vi "Handle Scroll.vi"(8 "error in (no error)":errorcluster, 9 "OldVal":i32, 10 "NewVal":i32, 11 "PanelArray in":refnum<class "PanelArray.lvclass">) -> (0 "error out":errorcluster, 3 "PanelArray out":refnum<class "PanelArray.lvclass">)   [LabVIEW 2018, in "OOPanel.lvlib" / "PanelArray.lvclass"]
uses:
  PanelArray.lvclass
  PanelArray.lvclass/PanelArray.ctl
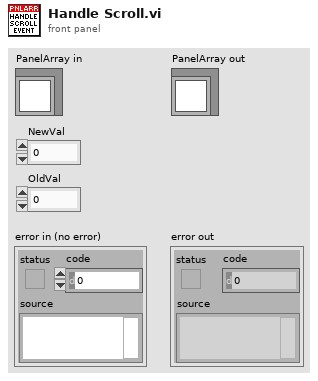
[diagram p1: front panel]
types:
  T1 = typedef "OOPanel.lvlib/PanelArray.lvclass/Ref Data.ctl" = cluster{"State":T2, "Refs":T3, "Events":T4, "Scrolling":T5, "Panels":T6}
  T2 = typedef "OOPanel.lvlib/PanelArray.lvclass/State.ctl" = cluster{"Defer Updates":bool, "Running":bool, "Dynamic Sizing":bool, "Borders":bool}
  T3 = typedef "OOPanel.lvlib/PanelArray.lvclass/Refs.ctl" = cluster{"SubPanels":refnum<vi>[], "Scrollbar":refnum<vi>, "Owning Panel":refnum<vi>}
  T4 = typedef "OOPanel.lvlib/PanelArray.lvclass/Events.ctl" = cluster{"Close":refnum<user-event>}
  T5 = typedef "OOPanel.lvlib/PanelArray.lvclass/Scrolling.ctl" = cluster{"Size":i32, "Max":i32, "Current":i32, "Top Index":i32, "Heights":i32[]}
  T6 = typedef "OOPanel.lvlib/PanelArray.lvclass/Panels.ctl" = cluster{"All":refnum<class "Panel.lvclass">[], "Visible":refnum<class "Panel.lvclass">[], "Blank":refnum<class "ArrayBlank.lvclass">}
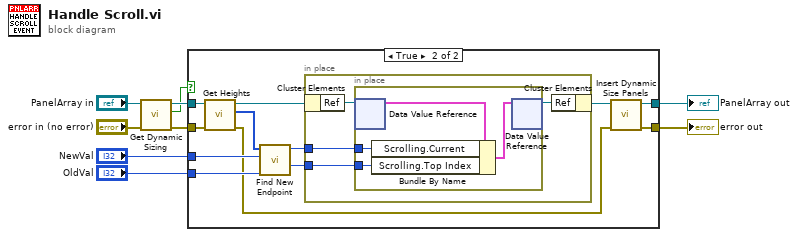
[diagram p0: block diagram]
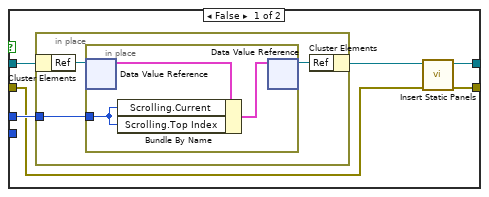
[diagram p2: hidden frame]
diagram:
  n1 = call "Get Dynamic Sizing.vi"("error in (no error)"="error in (no error)", "PanelArray in"="PanelArray in") -> ("error out"=w6:errorcluster, "Dynamic Sizing"=w3:bool, "PanelArray out"=w7:refnum<class "PanelArray.lvclass">)  [unwired: 7 in]
  n2 = case shown="True" w3 {
    tunnel: w7 -> [w15 w33]
    tunnel: w6 -> [w10 w32]
    tunnel: "NewVal" -> [w14 w30]
    tunnel: "OldVal" -> [_ w29]
    tunnel: [w12 w24] -> w2
    tunnel: [w13 w23] -> w1
    frame False {
      n3 = in-place {
        in-place-border: w14 -> [w17]
        n4 = in-place-cluster #1(w15) -> ("Ref"=w18:refnum<data-value>)
        n5 = in-place {
          in-place-border: w17 -> [w19]
          n6 = in-place-dvr #2(w18) -> (w21:T1)  [unwired: 1 out]
          n7 = Bundle By Name(cluster=w21, "Scrolling.Current"=w19, "Scrolling.Top Index"=w19) -> (w20:T1)
          n8 = in-place-dvr #2(w20) -> (w16:refnum<data-value>)  [unwired: 1 out]
        }
        n9 = in-place-cluster #1("Ref"=w16) -> (w11:refnum<class "PanelArray.lvclass">)
      }
      n10 = call "Insert Static Panels.vi"("error in (no error)"=w10, "PanelArray in"=w11) -> ("error out"=w13:errorcluster, "PanelArray out"=w12:refnum<class "PanelArray.lvclass">)  [unwired: 8 in]
    }
    frame True {
      n11 = call "Get Heights.vi"("error in (no error)"=w32, "PanelArray in"=w33) -> ("error out"=w22:errorcluster, "Heights"=w31:i32[], "PanelArray out"=w26:refnum<class "PanelArray.lvclass">)  [unwired: 7 in]
      n12 = call "Find New Endpoint.vi"("OldVal"=w29, "NewVal"=w30, "Heights"=w31) -> ("Index"=w27:i32, "Endpoint"=w28:i32)  [unwired: 7 in]
      n13 = in-place {
        in-place-border: w28 -> [w37]
        in-place-border: w27 -> [w36]
        n14 = in-place-cluster #3(w26) -> ("Ref"=w35:refnum<data-value>)
        n15 = in-place {
          in-place-border: w37 -> [w39]
          in-place-border: w36 -> [w38]
          n16 = in-place-dvr #4(w35) -> (w41:T1)  [unwired: 1 out]
          n17 = Bundle By Name(cluster=w41, "Scrolling.Current"=w39, "Scrolling.Top Index"=w38) -> (w40:T1)
          n18 = in-place-dvr #4(w40) -> (w34:refnum<data-value>)  [unwired: 1 out]
        }
        n19 = in-place-cluster #3("Ref"=w34) -> (w25:refnum<class "PanelArray.lvclass">)
      }
      n20 = call "Insert Dynamic Size Panels.vi"("error in (no error)"=w22, "PanelArray in"=w25) -> ("error out"=w23:errorcluster, "PanelArray out"=w24:refnum<class "PanelArray.lvclass">)  [unwired: 8 in]
    }
  }
  "error out" <- w1
  "PanelArray out" <- w2
